vi "CONVERT-TAG-SIGNAL-IO-NAME.vi"(4 "tag":string) -> (1 "signal":string)   [LabVIEW 2015]
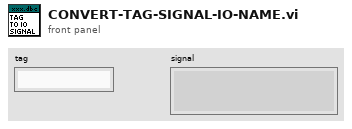
[diagram p1: front panel]
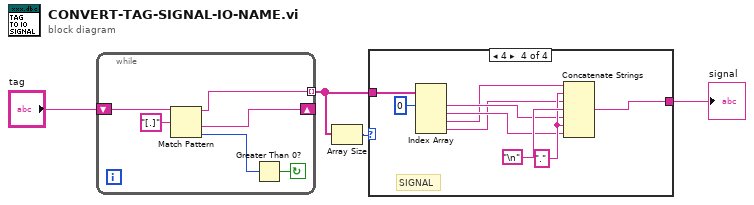
[diagram p0: block diagram]
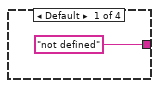
[diagram p2: hidden frame]
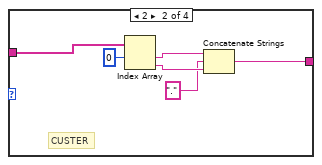
[diagram p3: hidden frame]
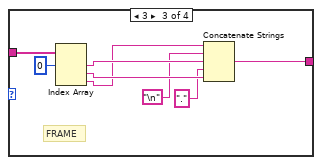
[diagram p4: hidden frame]
diagram:
  n1 = while {
    shift-right: [w9] -> _
    shift-left: "tag" -> [w10]
    tunnel: [w6] -> w2 mode=indexing
    stop <- w7 continue-if-true
    n2 = Match Pattern(string=w10, regular expression="[.]") -> (before substring=w6:string, after substring=w9:string, offset past match=w8:i32)  [unwired: 1 in, 1 out]
    n3 = Greater Than 0?(x=w8) -> (x > 0?=w7:bool)
  }
  n4 = Array Size(array=w2) -> (size(s)=w3:i32)
  n5 = case shown="4" w3 {
    tunnel: w2 -> [_ w17 w25 w32]
    tunnel: ["not defined" w13 w21 w28] -> w1
    frame Default {
    }
    frame 2 {
      # "CUSTER"
      n6 = Index Array(array=w17, index #1=0 ("index")) -> (element #1=w15:string, element #2=w14:string)  [unwired: 1 in]
      n7 = Concatenate Strings(w15, ".", w14) -> (w13:string)
    }
    frame 3 {
      # "FRAME"
      n8 = Index Array(array=w25, index #1=0 ("index")) -> (element #1=w23:string, element #2=w22:string, element #3=w19:string)  [unwired: 2 in]
      n9 = Concatenate Strings(w19, "\n", w23, ".", w22) -> (w21:string)
    }
    frame 4 {
      w33 = "."
      # "SIGNAL"
      n10 = Index Array(array=w32, index #1=0 ("index")) -> (element #1=w30:string, element #2=w29:string, element #3=w27:string, element #4=w26:string)  [unwired: 3 in]
      n11 = Concatenate Strings(w27, w33, w26, "\n", w30, w33, w29) -> (w28:string)
    }
  }
  "signal" <- w1
